vi "Wait Single Element Notification.vi"(8 "error in (no error)":errorcluster, 9 "Timeout":i32=-1, 11 "Notifier in":refnum<class "Notifier.lvclass">) -> (0 "error out":errorcluster, 1 "Timeout?":bool, 2 "I64 Notification":i64, 3 "Notifier out":refnum<class "Notifier.lvclass">, 4 "String":string, 6 "DBL Notification":dbl)   [LabVIEW 2024, in "Notifier.lvclass"]
uses:
  Notifier.lvclass
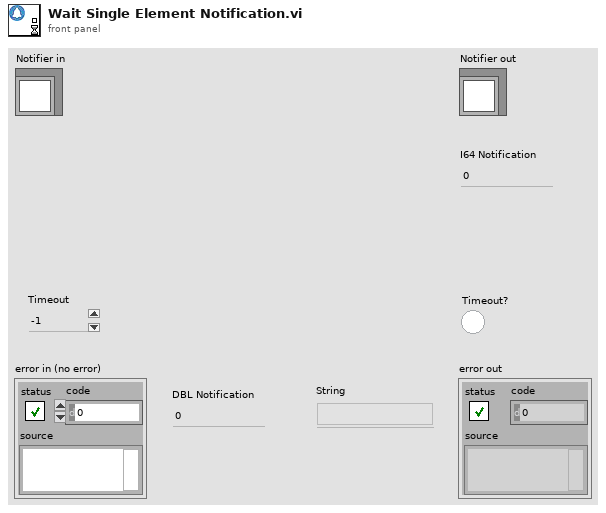
[diagram p1: front panel]
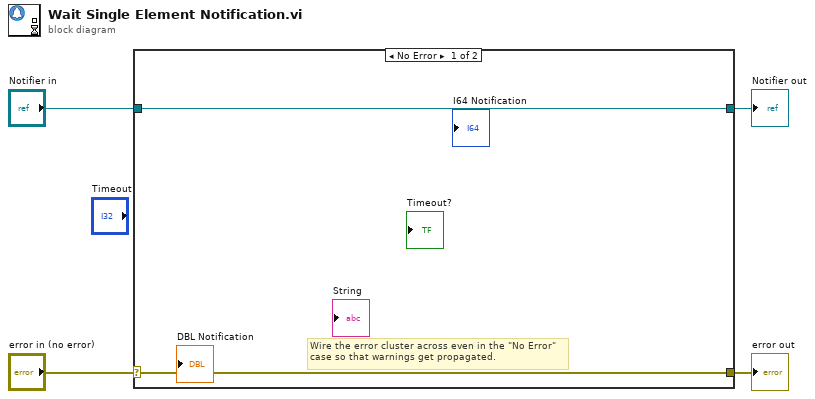
[diagram p0: block diagram]
diagram:
  n1 = case shown="No Error" "error in (no error)" {
    selector: "error in (no error)" -> [w5 w8]
    tunnel: [w5 w8] -> w3
    tunnel: [w6 w7] -> w1
    tunnel: "Notifier in" -> [w6 w7]
    frame No Error {
      # "Wire the error cluster across even in the \"No Error\"\ncase so that warnings get propagated."
    }
    frame Error {
    }
  }
  "error out" <- w3
  "Notifier out" <- w1
